vi "Teleop.vi"(10 "Match Info":T1={"Autonomous Elapsed Seconds"=0.0, "TeleOp Elapsed Seconds"=0.0, "Disabled Elapsed Seconds"=0.0, "Visited Autonomous"=FALSE, "Visited TeleOp"=FALSE, "Visited Disabled"=FALSE, "Autonomous Settings"={"Autonomous Style"=enum."Independent", "VI Refnum"=refnum}}, 11 "Call Context":T2) -> ()   [LabVIEW 2013]
doc: "This VI is called for each TeleOp packet received from the DS where the robot is not disabled. It is often used to read from the joysticks and update I/O or to update setpoints for timed control loops. It should complete and return within 20 milliseconds or it may miss DS packets."
uses:
  <vilib>/Rock Robotics/WPI/DriverStation/WPI_DriverStationDerivedRobotMode.ctl
  <vilib>/Rock Robotics/WPI/DriverStation/WPI_DriverStationMatch Info.ctl
  <vilib>/Rock Robotics/WPI/Solenoid/WPI_SolenoidValue.ctl
  Robot Global Data.vi
  <vilib>/Rock Robotics/WPI/Solenoid/Deprecated/WPI_SolenoidGetBool.vi
  <vilib>/Rock Robotics/WPI/Solenoid/WPI_SolenoidSetEnum.vi
  <vilib>/Rock Robotics/WPI/Joystick/WPI_JoystickGetSetRefNum.vi
  <vilib>/Rock Robotics/WPI/RobotDrive/WPI_RobotDriveGetSetRefNum.vi
panel:
  out "Numeric 1":dbl(slide) scale=0.0..100.0
  out "Boolean 2":bool
  out "Boolean 1":bool
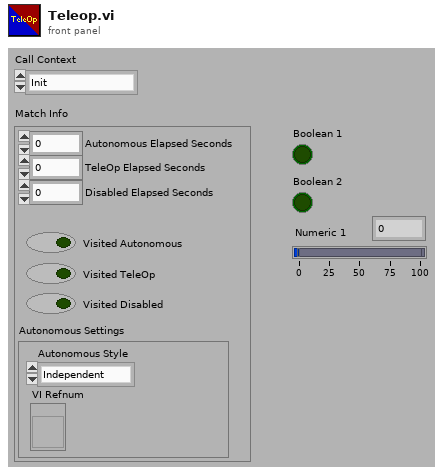
[diagram p1: front panel]
types:
  T1 = typedef "WPI_DriverStationMatch Info.ctl" = cluster{"Autonomous Elapsed Seconds":dbl, "TeleOp Elapsed Seconds":dbl, "Disabled Elapsed Seconds":dbl, "Visited Autonomous":bool, "Visited TeleOp":bool, "Visited Disabled":bool, "Autonomous Settings":cluster{"Autonomous Style":enum16{"Iterative", "Independent"}, "VI Refnum":refnum<vi>}}
  T2 = typedef "WPI_DriverStationDerivedRobotMode.ctl" = enum16{"Init", "Execute", "Stop"}
  T3 = typedef "WPI_RobotDriveDevRef.ctl" = cluster{"DevStatus":errorcluster, "Motors[]":T4[], "Square Inputs":bool, "Max Output":dbl, "Isochronous":bool}
  T4 = typedef "WPI_MotorControlDeviceRef.ctl" = cluster{"DeviceStatus":errorcluster, "Type":enum16{"PWM", "CAN"}, "PWM":cluster{"Digital Module":T5, "PWM Channel":T6, "DeadBand":T7}, "CAN":cluster{"Device Number":u8, "Control Mode":T8, "Semaphore":T9, "Max Vout":dbl}, "Invert":bool, "TransformRef":T10, "InvTransformRef":T10}
  T5 = typedef "FPGA_TypedefDigitalModule.ctl" = enum16{"Digital Module 1", "Digital Module 2"}
  T6 = typedef "FPGA_DIOPWMChannel.ctl" = enum8{"PWM 1", "PWM 2", "PWM 3", "PWM 4", "PWM 5", "PWM 6", "PWM 7", "PWM 8", "PWM 9", "PWM 10", "Invalid"}
  T7 = typedef "WPI_PWMDeadband.ctl" = cluster{"Name":string, "maxPositivePwm":i32, "minPositivePwm":i32, "centerPwm":i32, "maxNegativePwm":i32, "minNegativePwm":i32, "angularRange":u16}
  T8 = typedef "WPI_CANJaguar_ControlMode.ctl" = enum8{"Percent VBus", "Current", "Speed", "Position", "Voltage"}
  T9 = typedef "Semaphore RefNum" = refnum<k1>
  T10 = typedef "WPI_PWMTransform_ConPane.ctl" = refnum<vi>
  T11 = typedef "WPI_JoystickDevRef.ctl" = cluster{"Device":T12}
  T12 = typedef "WPI_JoystickDeviceEnum.ctl" = enum16{"USB 1", "USB 2", "USB 3", "USB 4", "Kinect 1", "Kinect 2"}
  T13 = typedef "WPI_JoystickButtonState.ctl" = cluster{"Button 1":bool, "Button 2":bool, "Button 3":bool, "Button 4":bool, "Button 5":bool, "Button 6":bool, "Button 7":bool, "Button 8":bool, "Button 9":bool, "Button 10":bool, "Button 11":bool, "Button 12":bool}
  T14 = cluster{"axis 1 (x)":dbl, "axis 2 (y)":dbl, "axis 3 (throttle)":dbl, "axis 4":dbl, "axis 5":dbl, "axis 6":dbl}
  T15 = typedef "WPI_AnalogChannelDevRef.ctl" = cluster{"DevStatus":errorcluster, "Analog Module":T16, "Analog Channel":T17}
  T16 = typedef "FPGA_TypedefAnalogModule.ctl" = enum16{"Analog Module 1", "Analog Module 2"}
  T17 = typedef "FPGA_AIChannel.ctl" = enum8{"AI 1", "AI 2", "AI 3", "AI 4", "AI 5", "AI 6", "AI 7", "AI 8", "Invalid"}
  T18 = typedef "WPI_RelayDevRef.ctl" = cluster{"DevStatus":errorcluster, "Relay Channel":T19, "Digital Module":T5, "Relay Direction":T20}
  T19 = typedef "FPGA_DIORelayChannel.ctl" = enum8{"Relay 1", "Relay 2", "Relay 3", "Relay 4", "Relay 5", "Relay 6", "Relay 7", "Relay 8", "Invalid"}
  T20 = typedef "WPI_RelayDirection.ctl" = enum16{"Both directions", "Forward only", "Reverse only"}
  T21 = typedef "WPI_SolenoidDevRef.ctl" = cluster{"DevStatus":errorcluster, "Solenoid Module":T22, "Forward Solenoid Channel":T23, "Reverse Solenoid Channel":T23}
  T22 = typedef "FPGA_TypedefSolenoidModule.ctl" = enum16{"Solenoid Module 1", "Solenoid Module 2"}
  T23 = typedef "WPI_SolenoidChannel.ctl" = enum8{"Solenoid 1", "Solenoid 2", "Solenoid 3", "Solenoid 4", "Solenoid 5", "Solenoid 6", "Solenoid 7", "Solenoid 8", "Invalid"}
  T24 = typedef "WPI_SolenoidValue.ctl" = enum16{"Off", "On", "Forward", "Reverse"}
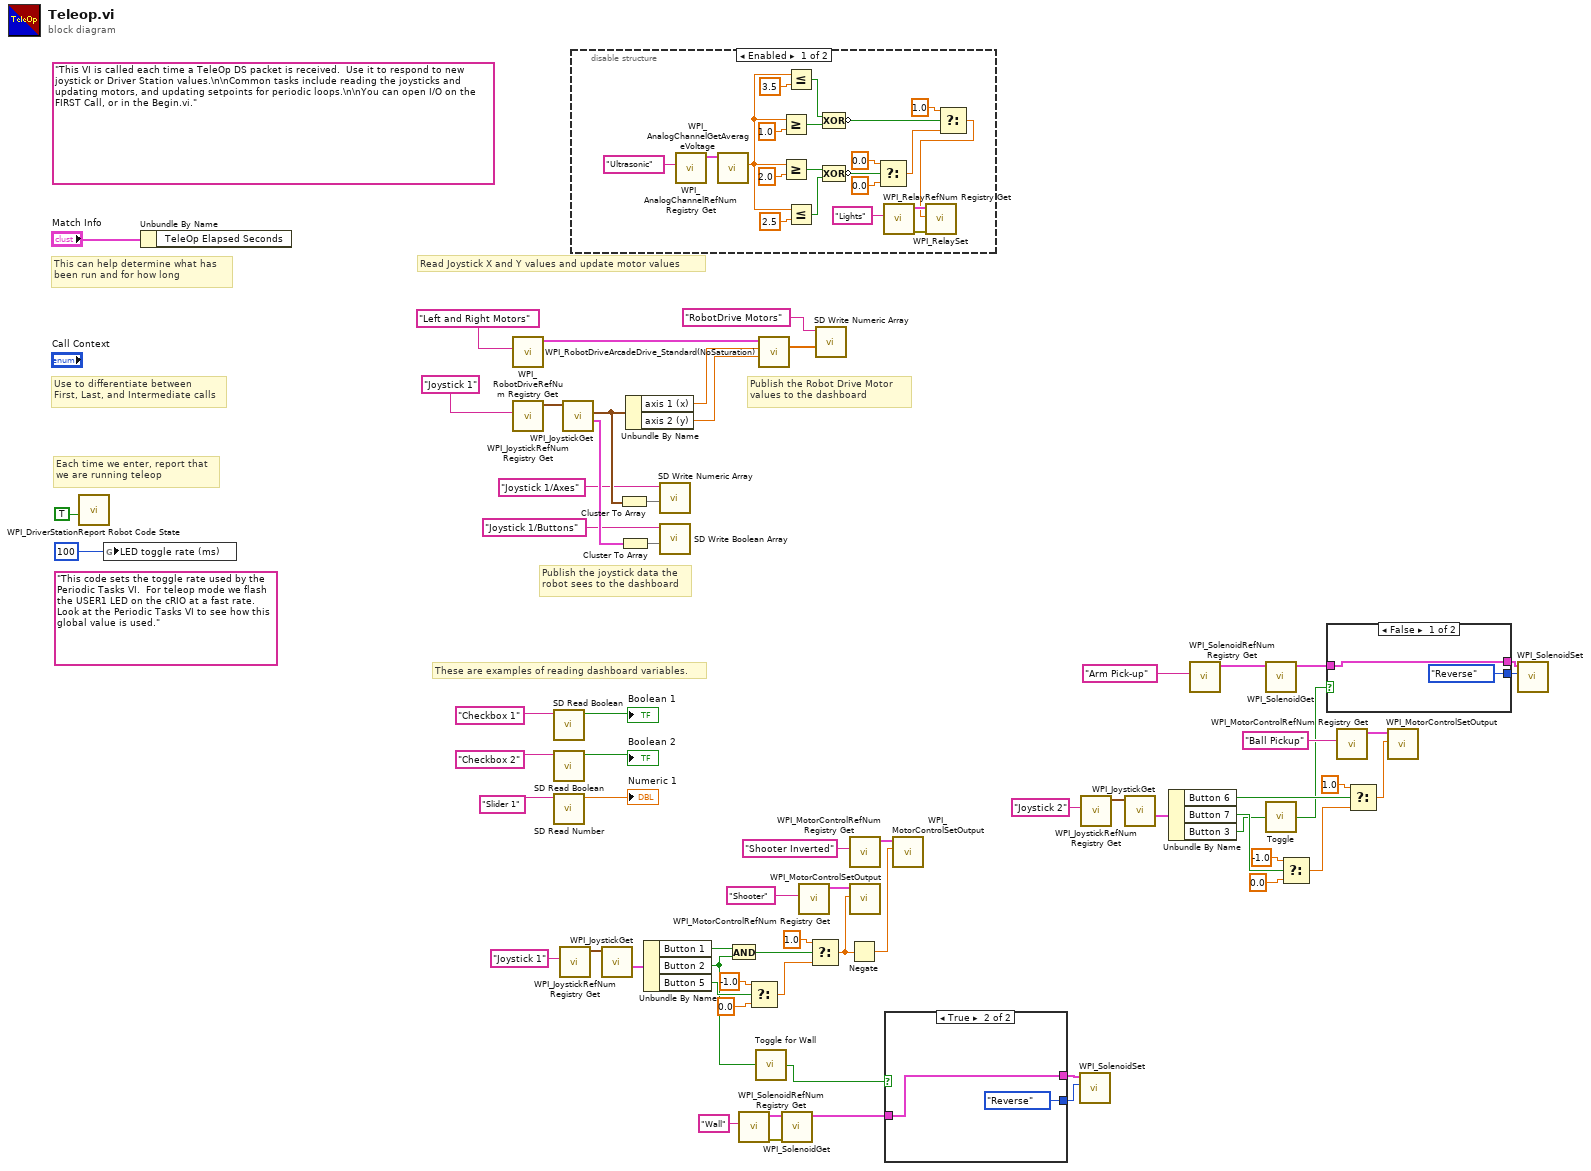
[diagram p0: block diagram]
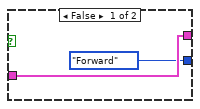
[diagram p2: hidden frame]
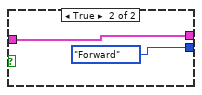
[diagram p4: hidden frame]
diagram:
  (unwired) "This code sets the toggle rate used by the Periodic Tasks VI.  For teleop mode we flash the USER1 LED on the cRIO at a fast rate.  Look at the Periodic Tasks VI to see how this global value is used."
  (unwired) "This VI is called each time a TeleOp DS packet is received.  Use it to respond to new joystick or Driver Station values.\n\nCommon tasks include reading the joysticks and updating motors, and updating setpoints for periodic loops.\n\nYou can open I/O on the FIRST Call, or in the Begin.vi."
  # "These are examples of reading dashboard variables."
  # "Publish the Robot Drive Motor\nvalues to the dashboard"
  # "Publish the joystick data the\nrobot sees to the dashboard"
  # "Each time we enter, report that\nwe are running teleop"
  # "Use to differentiate between\nFirst, Last, and Intermediate calls"
  # "This can help determine what has\nbeen run and for how long"
  # "Read Joystick X and Y values and update motor values"
  n1 = call <vilib>:"WPI_DriverStationReport Robot Code State.vi"("TeleOp"=TRUE ("Autonomous")) -> ()  [unwired: 10 in, 1 out]
  n2 = global write "Robot Global Data.vi" "LED toggle rate (ms)"(u32 100 ("LED ms toggle rate")) -> ()
  n3 = Unbundle By Name("Match Info") -> ()  [unwired: 1 out]
  n4 = call <vilib>:"WPI_RobotDriveRefNum Registry Get.vi"("refnum name"="Left and Right Motors") -> ("RobotDriveDevRef"=w64:T3)  [unwired: 1 in, 9 out]
  n5 = call <vilib>:"WPI_JoystickRefNum Registry Get.vi"("refnum name"="Joystick 1") -> ("JoystickDevRef"=w60:T11)  [unwired: 1 in, 9 out]
  n6 = call <vilib>:"SD Read Boolean.vi"("Name"="Checkbox 1" ("refnum name")) -> ("Boolean"=→"Boolean 1":bool)  [unwired: 8 in, 2 out]
  n7 = call <vilib>:"SD Read Boolean.vi"("Name"="Checkbox 2" ("refnum name")) -> ("Boolean"=→"Boolean 2":bool)  [unwired: 8 in, 2 out]
  n8 = call <vilib>:"SD Read Number.vi"("Name"="Slider 1" ("refnum name")) -> ("Numeric"=→"Numeric 1":dbl)  [unwired: 8 in, 2 out]
  n9 = call <vilib>:"WPI_JoystickRefNum Registry Get.vi"("refnum name"="Joystick 1") -> ("JoystickDevRef"=w42:T11)  [unwired: 1 in, 9 out]
  n10 = call <vilib>:"WPI_JoystickGet.vi"("JoystickDevRef"=w60) -> ("Buttons"=w57:T13, "Axes"=w54:T14)  [unwired: 1 in, 4 out]
  n11 = disable-structure shown="Enabled" {
    frame Enabled {
      n12 = call <vilib>:"WPI_AnalogChannelRefNum Registry Get.vi"("refnum name"="Ultrasonic") -> ("AIDeviceRef"=w86:T15)  [unwired: 9 in, 1 out]
      n13 = call <vilib>:"WPI_AnalogChannelGetAverageVoltage.vi"("AIDeviceRef"=w86) -> ("Voltage"=w77:dbl)  [unwired: 8 in, 2 out]
      n14 = Greater Or Equal?(x=w77, y=1.0) -> (x >= y?=w80:bool)
      n15 = Greater Or Equal?(x=w77, y=2.0) -> (x >= y?=w74:bool)
      n16 = Less Or Equal?(x=w77, y=3.5) -> (x <= y?=w79:bool)
      n17 = Less Or Equal?(x=w77, y=2.5) -> (x <= y?=w75:bool)
      n18 = Compound Arithmetic op=XOR(w79, w80) -> (invert w72:bool)
      n19 = Compound Arithmetic op=XOR(w74, w75) -> (invert w73:bool)
      n20 = Select(t=0.0, s=w73, f=0.0) -> (s? t:f=w68:dbl)
      n21 = call <vilib>:"WPI_RelayRefNum Registry Get.vi"("refnum name"="Lights") -> ("error out"=w85:errorcluster, "RelayDevRef"=w84:T18)  [unwired: 9 in]
      n22 = Select(t=1.0, s=w72, f=w68) -> (s? t:f=w67:dbl)
      n23 = call <vilib>:"WPI_RelaySet.vi"("error in (no error)"=w85, "RelayValue"=w67, "RelayDevRef"=w84) -> ()  [unwired: 7 in, 2 out]
    }
    frame Disabled {
    }
  }
  n24 = call <vilib>:"WPI_JoystickGet.vi"("JoystickDevRef"=w42) -> ("Buttons"=w41:T13)  [unwired: 1 in, 5 out]
  n25 = Cluster To Array(cluster=w54) -> (array=w53:dbl[])
  n26 = Cluster To Array(cluster=w57) -> (array=w56:bool[])
  n27 = Unbundle By Name(w54) -> ("axis 1 (x)"=w63:dbl, "axis 2 (y)"=w62:dbl)
  n28 = Unbundle By Name(w41) -> ("Button 1"=w40:bool, "Button 2"=w8:bool, "Button 5"=w38:bool)
  n29 = call <vilib>:"SD Write Numeric Array.vi"("Numeric Array"=w53, "Name"="Joystick 1/Axes") -> ()  [unwired: 8 in, 2 out]
  n30 = call <vilib>:"SD Write Boolean Array.vi"("Boolean Array"=w56, "Name"="Joystick 1/Buttons") -> ()  [unwired: 8 in, 2 out]
  n31 = And(x=w40, y=w8) -> (x .and. y?=w39:bool)
  n32 = call <vilib>:"WPI_SolenoidRefNum Registry Get.vi"("refnum name"="Wall") -> ("error out"=w10:errorcluster, "SolenoidDevRef"=w9:T21)  [unwired: 9 in]
  n33 = Select(t=-1.0, s=w38, f=0.0) -> (s? t:f=w34:dbl)
  n34 = call "Toggle for Wall.vi"("Input"=w8) -> ("Toggled Output"=w7:bool)
  n35 = call <vilib>:"WPI_RobotDriveArcadeDrive_Standard(NoSaturation).vi"("Y axis value"=w62, "X axis value"=w63, "RobotDriveDevRef"=w64) -> ("Motor Values"=w50:dbl[])  [unwired: 1 in, 7 out]
  n36 = call-poly <vilib>:"WPI_SolenoidGet.vi"("error in (no error)"=w10, "SolenoidDevRef"=w9) -> ("SolenoidDevRef"=w4:T21)  [unwired: 7 in, 2 out]
  n37 = call <vilib>:"WPI_MotorControlRefNum Registry Get.vi"("refnum name"="Shooter") -> ("MotorControlDevRef"=w32:T4)  [unwired: 9 in, 1 out]
  n38 = Select(t=1.0, s=w39, f=w34) -> (s? t:f=w31:dbl)
  n39 = call <vilib>:"SD Write Numeric Array.vi"("Numeric Array"=w50, "Name"="RobotDrive Motors") -> ()  [unwired: 8 in, 2 out]
  n40 = Negate(x=w31) -> (-x=w29:dbl)
  n41 = call <vilib>:"WPI_MotorControlRefNum Registry Get.vi"("refnum name"="Shooter Inverted") -> ("MotorControlDevRef"=w28:T4)  [unwired: 9 in, 1 out]
  n42 = call <vilib>:"WPI_MotorControlSetOutput.vi"("Output"=w31, "MotorControlDevRef"=w32) -> ()  [unwired: 7 in, 3 out]
  n43 = case shown="True" w7 {
    tunnel: w4 -> [w89 w91]
    tunnel: [w89 w91] -> w3
    tunnel: [WPI_SolenoidValue."Forward" ("Value") WPI_SolenoidValue."Reverse" ("Value")] -> w2
    frame False {
    }
    frame True {
    }
  }
  n44 = call <vilib>:"WPI_MotorControlSetOutput.vi"("Output"=w29, "MotorControlDevRef"=w28) -> ()  [unwired: 7 in, 3 out]
  n45 = call-poly <vilib>:"WPI_SolenoidSet.vi"("Value"=w2, "SolenoidDevRef"=w3) -> ()  [unwired: 8 in, 2 out]
  n46 = call <vilib>:"WPI_JoystickRefNum Registry Get.vi"("refnum name"="Joystick 2") -> ("JoystickDevRef"=w27:T11)  [unwired: 1 in, 9 out]
  n47 = call <vilib>:"WPI_JoystickGet.vi"("JoystickDevRef"=w27) -> ("Buttons"=w25:T13)  [unwired: 1 in, 5 out]
  n48 = Unbundle By Name(w25) -> ("Button 6"=w23:bool, "Button 7"=w24:bool, "Button 3"=w15:bool)
  n49 = call <vilib>:"WPI_SolenoidRefNum Registry Get.vi"("refnum name"="Arm Pick-up") -> ("SolenoidDevRef"=w13:T21)  [unwired: 9 in, 1 out]
  n50 = call-poly <vilib>:"WPI_SolenoidGet.vi"("SolenoidDevRef"=w13) -> ("SolenoidDevRef"=w12:T21)  [unwired: 8 in, 2 out]
  n51 = call "Toggle.vi"("Input"=w15) -> ("Toggled Output"=w14:bool)
  n52 = Select(t=-1.0, s=w24, f=0.0) -> (s? t:f=w19:dbl)
  n53 = case shown="False" w14 {
    tunnel: w12 -> [w93 w95]
    tunnel: [w93 w95] -> w6
    tunnel: [WPI_SolenoidValue."Reverse" ("Value") WPI_SolenoidValue."Forward" ("Value")] -> w5
    frame False {
    }
    frame True {
    }
  }
  n54 = call <vilib>:"WPI_MotorControlRefNum Registry Get.vi"("refnum name"="Ball Pickup") -> ("MotorControlDevRef"=w17:T4)  [unwired: 9 in, 1 out]
  n55 = Select(t=1.0, s=w23, f=w19) -> (s? t:f=w16:dbl)
  n56 = call <vilib>:"WPI_MotorControlSetOutput.vi"("Output"=w16, "MotorControlDevRef"=w17) -> ()  [unwired: 7 in, 3 out]
  n57 = call-poly <vilib>:"WPI_SolenoidSet.vi"("Value"=w5, "SolenoidDevRef"=w6) -> ()  [unwired: 8 in, 2 out]
